vi "DAC Init Results.vi"(8 "error in":errorcluster, 9 "Log Details?":bool, 10 "tdms file":refnum<k34>, 11 "DAC HeatFlow AIV in":refnum<class "DAC HeatFlow AOV.lvclass">) -> (0 "error out":errorcluster, 2 "tdms file out":refnum<k34>)   [LabVIEW 2019, in "DAC.lvlib" / "DAC HeatFlow AOV.lvclass"]
uses:
  DAC HeatFlow AOV.lvclass
  C:/Users/krio/Documents/LV_Projects/test-stand/App/DAC/DAC.lvclass
  DAC.lvclass/DAC.ctl
  DAC HeatFlow AOV.lvclass/DAC HeatFlow AOV.ctl
  DAC.lvclass
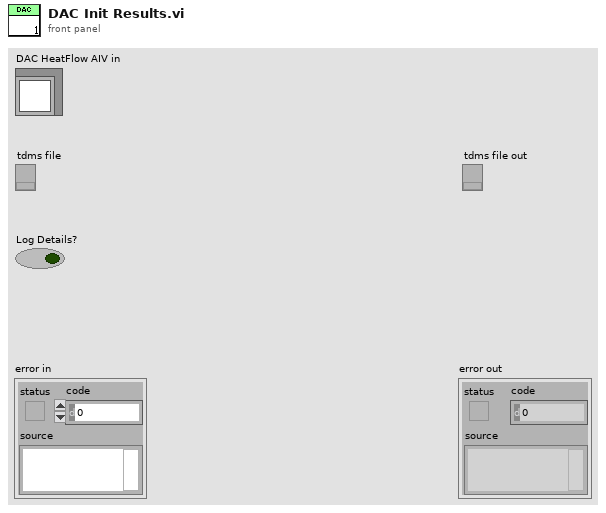
[diagram p1: front panel]
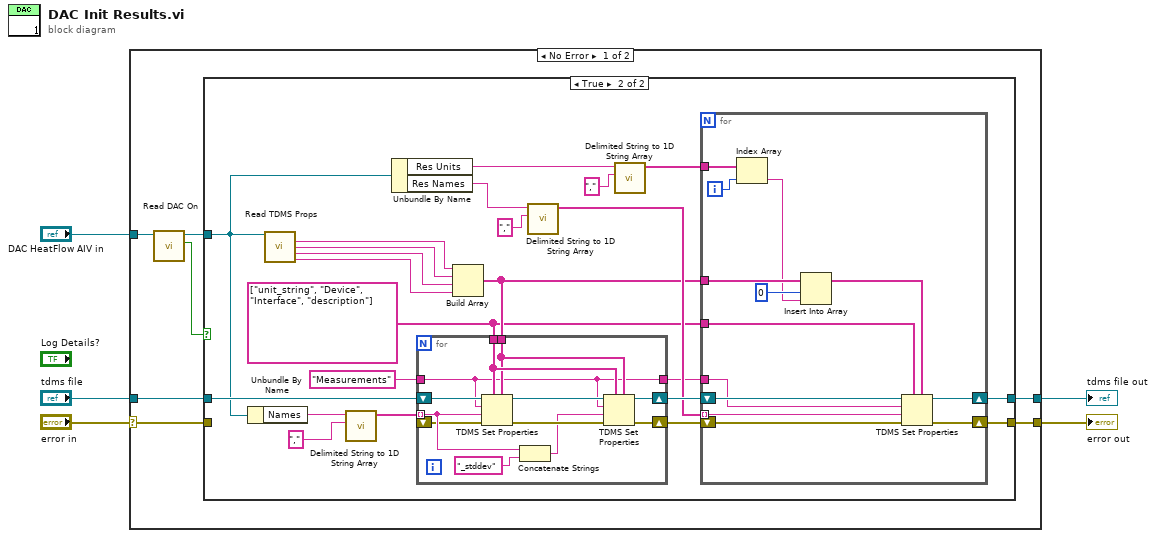
[diagram p0: block diagram]
diagram:
  n1 = case shown="No Error" "error in" {
    selector: "error in" -> [w7 w64]
    tunnel: [w10 w64] -> w2
    tunnel: "DAC HeatFlow AIV in" -> [w9 _]
    tunnel: "tdms file" -> [w12 w63]
    tunnel: [w11 w63] -> w1
    frame No Error {
      n2 = call "Read DAC On.vi"("DAC in"=w9) -> ("DAC On"=w6:bool, "DAC out"=w8:refnum<class "DAC HeatFlow AOV.lvclass">)  [unwired: 8 in, 1 out]
      n3 = case shown="True" w6 {
        tunnel: w12 -> [w14 w37]
        tunnel: [w14 w27] -> w11
        tunnel: [w13 w25] -> w10
        tunnel: w8 -> [_ w24]
        tunnel: w7 -> [w13 _]
        frame False {
        }
        frame True {
          w15 = string[] ["unit_string", "Device", "Interface", "description"] ("property names")
          n4 = Unbundle By Name(w24) -> ("Names"=w34:string)
          n5 = call "Read TDMS Props.vi"("DAC in"=w24) -> ("Result Unit"=w33:string, "DAC Device"=w32:string, "DAC IO"=w31:string, "DAC Description"=w30:string)  [unwired: 10 in, 1 out]
          n6 = call <vilib>:"Delimited String to 1D String Array.vi"("delimiter"=",", "delimited string"=w34) -> ("string array"=w36:string[])  [unwired: 9 in]
          n7 = Unbundle By Name(w24) -> ("Res Units"=w19:string, "Res Names"=w22:string)
          n8 = Build Array(w33, w32, w31, w30) -> (w17:string[])
          n9 = for {
            tunnel: w36 -> [w54] mode=indexing
            tunnel: w15 -> [w57]
            tunnel: w17 -> [w56]
            shift-right: [w58] -> w28
            shift-left: w37 -> [w62]
            tunnel: "Measurements" ("group name in (Untitled)") -> [w51]
            shift-right: [w60] -> w26
            shift-left: _ -> [w52]
            tunnel: [w51] -> w16
            n10 = TDMS Set Properties(5:w56, 7:w57, 8:w52, 9:w54, 10:w51, 11:w62) -> (0:w61:errorcluster, 3:w59:refnum<k34>)  [unwired: 2 out]
            n11 = Concatenate Strings(w54, "_stddev" ("string")) -> (w53:string)
            n12 = TDMS Set Properties(5:w56, 7:w57, 8:w61, 9:w53, 10:w51, 11:w59) -> (0:w60:errorcluster, 3:w58:refnum<k34>)  [unwired: 2 out]
          }
          n13 = call <vilib>:"Delimited String to 1D String Array.vi"("delimiter"=",", "delimited string"=w22) -> ("string array"=w21:string[])  [unwired: 9 in]
          n14 = call <vilib>:"Delimited String to 1D String Array.vi"("delimiter"=",", "delimited string"=w19) -> ("string array"=w18:string[])  [unwired: 9 in]
          n15 = for {
            shift-right: [w49] -> w27
            shift-left: w28 -> [w50]
            shift-right: [w47] -> w25
            shift-left: w26 -> [w48]
            tunnel: w21 -> [w46] mode=indexing
            tunnel: w18 -> [w44]
            tunnel: w17 -> [w42]
            tunnel: w16 -> [w45]
            tunnel: w15 -> [w39]
            i -> [w43]
            n16 = Index Array "Index Array"(array=w44, index=w43) -> (element=w40:string)
            n17 = Insert Into Array "Insert Into Array"(array=w42, index=0, new element=w40) -> (w38:string[])
            n18 = TDMS Set Properties(5:w38, 7:w39, 8:w48, 9:w46, 10:w45, 11:w50) -> (0:w47:errorcluster, 3:w49:refnum<k34>)  [unwired: 2 out]
          }
        }
      }
    }
    frame Error {
    }
  }
  "error out" <- w2
  "tdms file out" <- w1
